vi "Get Value.vi"(8 "error in (no error)":errorcluster, 11 "DA Parent in":refnum<class "DA Parent.lvclass">) -> (0 "error out":errorcluster, 2 "Value":string, 3 "DA Parent out":refnum<class "DA Parent.lvclass">)   [LabVIEW 2020, in "Display As.lvlib" / "DA Parent.lvclass"]
uses:
  DA Parent.lvclass
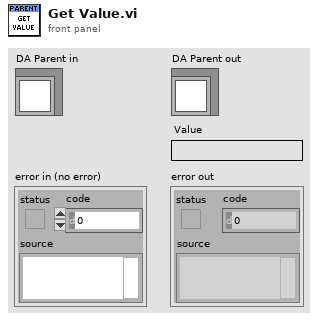
[diagram p1: front panel]
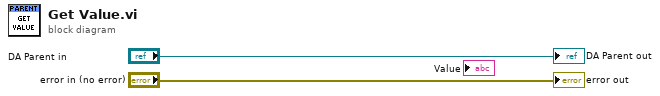
[diagram p0: block diagram]
diagram:
  "error out" <- "error in (no error)"
  "DA Parent out" <- "DA Parent in"
